vi "new.uxx.be.vi"(0 "buffer (U64)":u64[](array[numeric])=[216465256531934122, 1234605616436508552, 0, 0, 0, 0, 0, 0, 0] format="%016x", 1 "Start.Idx":u8, 2 "Length":u8=2, 3 "Big.Endian?":bool) -> (7 "Out.Value U64":u64 format="%.0x")   [LabVIEW 2020]
panel:
  out "Final Word":u64 format="%.0x"
  out "U32.le":u32 format="%.0x"
  out "U16.le":u16 format="%.0x"
  out "U8.le":u8 format="%.0x"
  out "Mask 3":u64 format="%016x"
  out "U8.be":u8 format="%.0x"
  out "16bit integer":i16 format="%.0x"
  out "# of bytes to extract":u8
  out "Second Word.Shifted":u64 format="%016x"
  out "U32.be":u32 format="%.0x"
  out "Second Word":u64 format="%016x"
  out "Mask 2":u64 format="%016x"
  out "Mask":u64 format="%016x"
  out "# of already valid bytes":u8
  out "Left Shift (in bits)":u8
  out "Left Shift (in bytes)":u8
  out "First.Word":u64 format="%016x"
  out "U16.be":u16 format="%.0x"
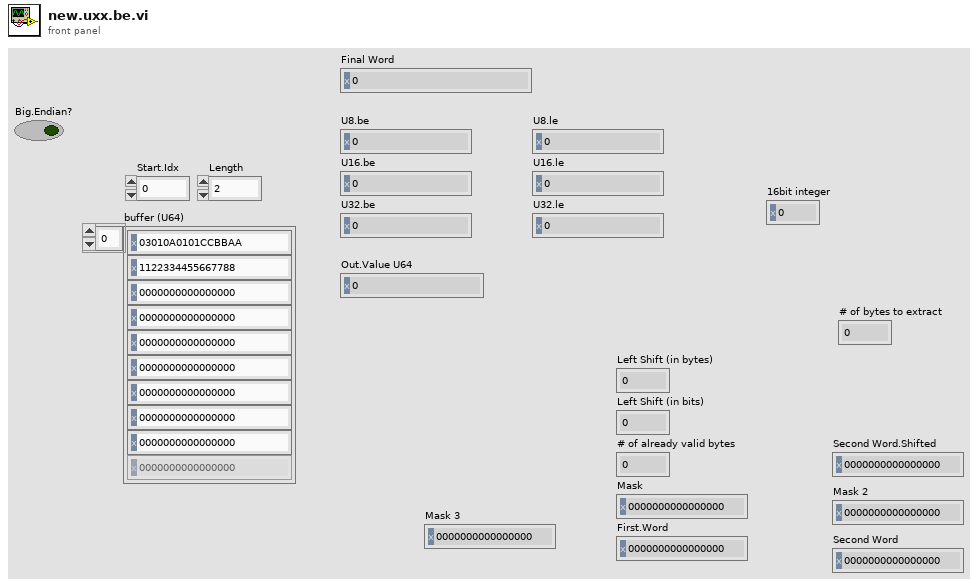
[diagram p1: front panel]
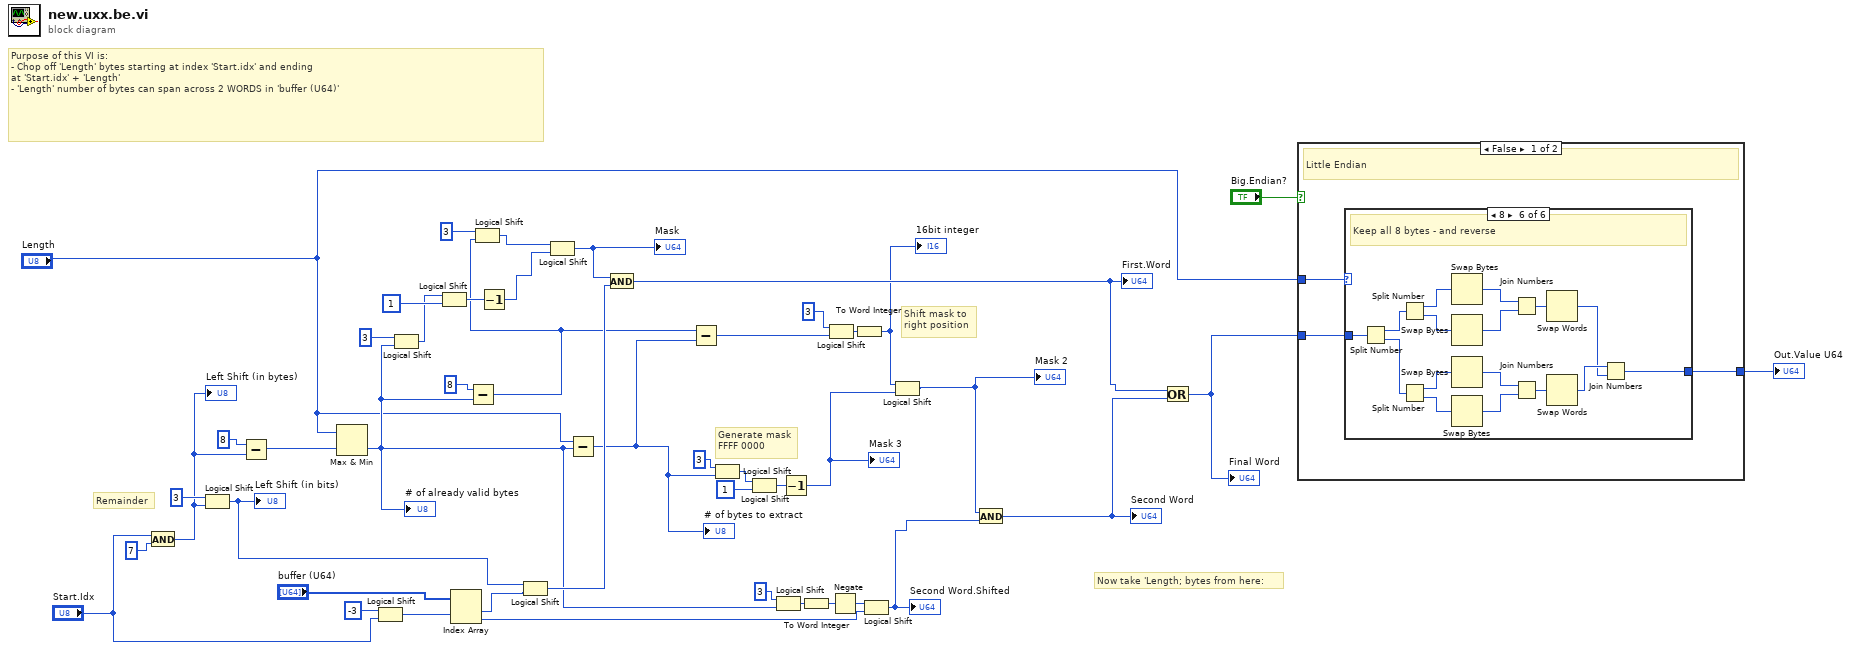
[diagram p0: block diagram]
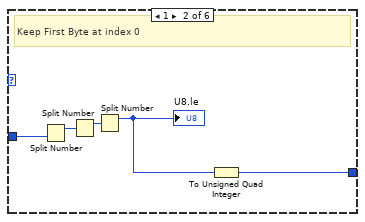
[diagram p3: hidden frame]
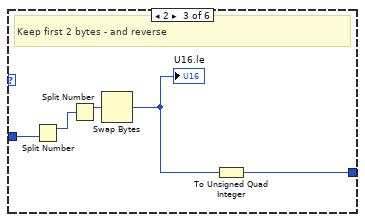
[diagram p4: hidden frame]
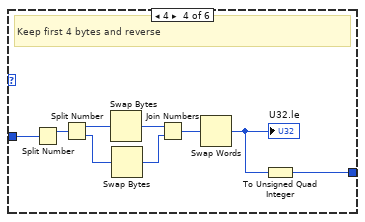
[diagram p5: hidden frame]
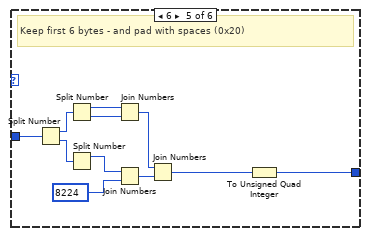
[diagram p6: hidden frame]
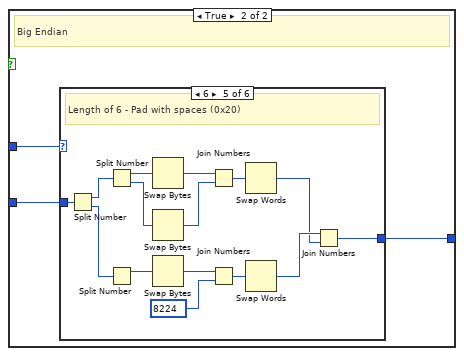
[diagram p7: hidden frame]
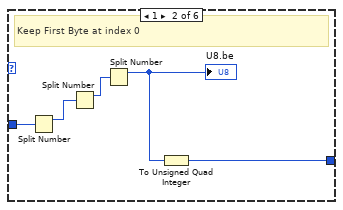
[diagram p9: hidden frame]
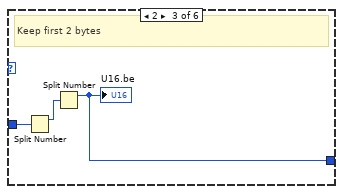
[diagram p10: hidden frame]
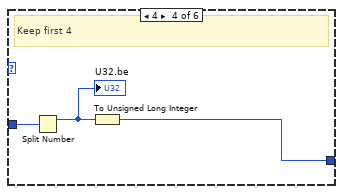
[diagram p11: hidden frame]
diagram:
  # "Now take 'Length; bytes from here:"
  # "Purpose of this VI is:\n- Chop off 'Length' bytes starting at index 'Start.idx' and ending\nat 'Start.idx' + 'Length'\n- 'Length' number of bytes can span across 2 WORDS in 'buffer (U64)'"
  # "Remainder"
  # "Shift mask to\nright position"
  # "Generate mask\nFFFF 0000"
  n1 = And(x="Start.Idx", y=u8 7 ("x")) -> (x .and. y?=w36:u8)
  "Left Shift (in bytes)" <- w36
  n2 = Logical Shift(y=i16 3, x=w36) -> (x << y=w29:u8)
  "Left Shift (in bits)" <- w29
  n3 = Subtract(x=u8 8, y=w36) -> (x-y=w39:u8)
  n4 = Max & Min(x="Length", y=w39) -> (min(x,y)=w13:u8)  [unwired: 1 out]
  "# of already valid bytes" <- w13
  n5 = Logical Shift(y=i16 -3, x="Start.Idx") -> (x << y=w30:u8)
  n6 = Logical Shift(y=i16 3, x=w13) -> (x << y=w40:u8)
  n7 = Logical Shift(y=w40, x=u64 1) -> (x << y=w42:u64)
  n8 = Index Array(array="buffer (U64)", index #1=w30) -> (element #1=w28:u64, element #2=w22:u64)  [unwired: 1 in]
  n9 = Subtract(x=u8 8, y=w13) -> (x-y=w3:u8)
  n10 = Logical Shift(y=i16 3, x=w3) -> (x << y=w37:u8)
  n11 = Decrement(x=w42) -> (x-1=w35:u64)
  n12 = Logical Shift(y=w29, x=w28) -> (x << y=w26:u64)
  n13 = Logical Shift(y=w37, x=w35) -> (x << y=w27:u64)
  "Mask" <- w27
  n14 = Subtract(x="Length", y=w13) -> (x-y=w2:u8)
  "# of bytes to extract" <- w2
  n15 = And(x=w27, y=w26) -> (x .and. y?=w17:u64)
  "First.Word" <- w17
  n16 = Subtract(x=w3, y=w2) -> (x-y=w8:u8)
  n17 = Logical Shift(y=i16 3, x=w2) -> (x << y=w21:u8)
  n18 = Logical Shift(y=w21, x=u64 1) -> (x << y=w24:u64)
  n19 = Logical Shift(y=i16 3, x=w13) -> (x << y=w4:u8)
  n20 = Decrement(x=w24) -> (x-1=w9:u64)
  "Mask 3" <- w9
  n21 = To Word Integer(number=w4) -> (16bit integer=w6:i16)
  n22 = Logical Shift(y=i16 3, x=w8) -> (x << y=w19:u8)
  n23 = Negate(x=w6) -> (-x=w7:i16)
  n24 = To Word Integer(number=w19) -> (16bit integer=w15:i16)
  "16bit integer" <- w15
  n25 = Logical Shift(y=w7, x=w22) -> (x << y=w14:u64)
  "Second Word.Shifted" <- w14
  n26 = Logical Shift(y=w15, x=w9) -> (x << y=w12:u64)
  "Mask 2" <- w12
  n27 = And(x=w12, y=w14) -> (x .and. y?=w18:u64)
  "Second Word" <- w18
  n28 = Or(x=w17, y=w18) -> (x .or. y?=w16:u64)
  "Final Word" <- w16
  n29 = case shown="False" "Big.Endian?" {
    tunnel: w16 -> [w48 w98]
    tunnel: "Length" -> [w49 w97]
    tunnel: [w47 w96] -> w10
    frame False {
      # "Little Endian"
      n30 = case shown="8" w49 {
        tunnel: w48 -> [_ w53 w58 w66 w78 w81]
        tunnel: [_ w50 w55 w60 w69 w80] -> w47
        frame 0, Default {
          # "Length of 0 -> Return 0"
        }
        frame 1 {
          # "Keep First Byte at index 0"
          n31 = Split Number(x=w53) -> (hi(x)=w54:u32)  [unwired: 1 out]
          n32 = Split Number(x=w54) -> (hi(x)=w52:u16)  [unwired: 1 out]
          n33 = Split Number(x=w52) -> (hi(x)=w51:u8)  [unwired: 1 out]
          "U8.le" <- w51
          n34 = To Unsigned Quad Integer(1:w51) -> (0:w50:u64)
        }
        frame 2 {
          # "Keep first 2 bytes - and reverse"
          n35 = Split Number(x=w58) -> (hi(x)=w59:u32)  [unwired: 1 out]
          n36 = Split Number(x=w59) -> (hi(x)=w57:u16)  [unwired: 1 out]
          n37 = Swap Bytes(anything=w57) -> (byte swapped=w56:u16)
          "U16.le" <- w56
          n38 = To Unsigned Quad Integer(1:w56) -> (0:w55:u64)
        }
        frame 4 {
          # "Keep first 4 bytes and reverse"
          n39 = Split Number(x=w66) -> (hi(x)=w68:u32)  [unwired: 1 out]
          n40 = Split Number(x=w68) -> (hi(x)=w67:u16, lo(x)=w65:u16)
          n41 = Swap Bytes(anything=w67) -> (byte swapped=w63:u16)
          n42 = Swap Bytes(anything=w65) -> (byte swapped=w62:u16)
          n43 = Join Numbers(hi=w63, lo=w62) -> ((hi.lo)=w64:u32)
          n44 = Swap Words(1:w64) -> (0:w61:u32)
          "U32.le" <- w61
          n45 = To Unsigned Quad Integer(1:w61) -> (0:w60:u64)
        }
        frame 6 {
          # "Keep first 6 bytes - and pad with spaces (0x20)"
          n46 = Split Number(x=w78) -> (hi(x)=w79:u32, lo(x)=w74:u32)
          n47 = Split Number(x=w79) -> (hi(x)=w72:u16, lo(x)=w77:u16)
          n48 = Split Number(x=w74) -> (hi(x)=w76:u16)  [unwired: 1 out]
          n49 = Join Numbers(hi=w72, lo=w77) -> ((hi.lo)=w73:u32)
          n50 = Join Numbers(hi=w76, lo=u16 8224 ("hi")) -> ((hi.lo)=w71:u32)
          n51 = Join Numbers(hi=w73, lo=w71) -> ((hi.lo)=w75:u64)
          n52 = To Unsigned Quad Integer(1:w75) -> (0:w69:u64)
        }
        frame 8 {
          # "Keep all 8 bytes - and reverse"
          n53 = Split Number(x=w81) -> (hi(x)=w95:u32, lo(x)=w84:u32)
          n54 = Split Number(x=w95) -> (hi(x)=w94:u16, lo(x)=w93:u16)
          n55 = Split Number(x=w84) -> (hi(x)=w89:u16, lo(x)=w88:u16)
          n56 = Swap Bytes(anything=w94) -> (byte swapped=w91:u16)
          n57 = Swap Bytes(anything=w93) -> (byte swapped=w90:u16)
          n58 = Swap Bytes(anything=w89) -> (byte swapped=w86:u16)
          n59 = Swap Bytes(anything=w88) -> (byte swapped=w85:u16)
          n60 = Join Numbers(hi=w91, lo=w90) -> ((hi.lo)=w92:u32)
          n61 = Join Numbers(hi=w86, lo=w85) -> ((hi.lo)=w87:u32)
          n62 = Swap Words(1:w92) -> (0:w82:u32)
          n63 = Swap Words(1:w87) -> (0:w83:u32)
          n64 = Join Numbers(hi=w83, lo=w82) -> ((hi.lo)=w80:u64)
        }
      }
    }
    frame True {
      # "Big Endian"
      n65 = case shown="6" w97 {
        tunnel: w98 -> [_ w102 w105 w109 w122 w125]
        tunnel: [_ w99 w104 w108 w112 w125] -> w96
        frame 0, Default {
          # "Length of 0 -> Return 0"
        }
        frame 1 {
          # "Keep First Byte at index 0"
          n66 = Split Number(x=w102) -> (hi(x)=w103:u32)  [unwired: 1 out]
          n67 = Split Number(x=w103) -> (hi(x)=w101:u16)  [unwired: 1 out]
          n68 = Split Number(x=w101) -> (hi(x)=w100:u8)  [unwired: 1 out]
          "U8.be" <- w100
          n69 = To Unsigned Quad Integer(1:w100) -> (0:w99:u64)
        }
        frame 2 {
          # "Keep first 2 bytes"
          n70 = Split Number(x=w105) -> (hi(x)=w106:u32)  [unwired: 1 out]
          n71 = Split Number(x=w106) -> (hi(x)=w104:u16)  [unwired: 1 out]
          "U16.be" <- w104
        }
        frame 4 {
          # "Keep first 4"
          n72 = Split Number(x=w109) -> (hi(x)=w107:u32)  [unwired: 1 out]
          "U32.be" <- w107
          n73 = To Unsigned Long Integer(number=w107) -> (unsigned 32bit integer=w108:u32)
        }
        frame 6 {
          # "Length of 6 - Pad with spaces (0x20)"
          n74 = Split Number(x=w122) -> (hi(x)=w124:u32, lo(x)=w115:u32)
          n75 = Split Number(x=w124) -> (hi(x)=w123:u16, lo(x)=w121:u16)
          n76 = Split Number(x=w115) -> (hi(x)=w117:u16)  [unwired: 1 out]
          n77 = Swap Bytes(anything=w123) -> (byte swapped=w119:u16)
          n78 = Swap Bytes(anything=w121) -> (byte swapped=w118:u16)
          n79 = Swap Bytes(anything=w117) -> (byte swapped=w111:u16)
          n80 = Join Numbers(hi=w119, lo=w118) -> ((hi.lo)=w120:u32)
          n81 = Join Numbers(hi=w111, lo=u16 8224 ("hi")) -> ((hi.lo)=w116:u32)
          n82 = Swap Words(1:w120) -> (0:w113:u32)
          n83 = Swap Words(1:w116) -> (0:w114:u32)
          n84 = Join Numbers(hi=w114, lo=w113) -> ((hi.lo)=w112:u64)
        }
        frame 8 {
          # "8 bytes ->Pass through"
        }
      }
    }
  }
  "Out.Value U64" <- w10
